vi "ParseObject.vi"(8 "error in (no error)":errorcluster, 10 "Index In":i32, 11 "JSON String":string) -> (0 "error out":errorcluster, 2 "Index Out":i32, 3 "JSON Tree":variant)   [LabVIEW 2013, in "i3-json.lvlib"]
doc: "Use this template to build a VI to use as a subVI."
uses:
  i3-json.lvlib
  JSON Types/JSON Type.ctl
  Token.ctl
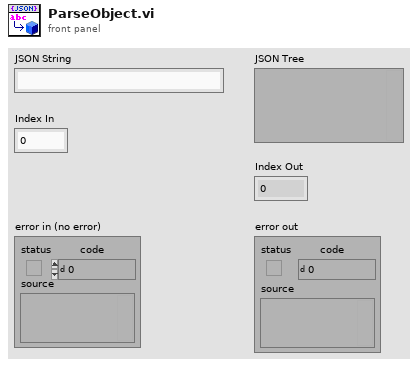
[diagram p1: front panel]
types:
  T1 = typedef "i3-json.lvlib/JSON Type.ctl" = enum8{"JSON Compatible", "JSON Array", "JSON Object", "JSON Null", "Double", "String", "Boolean", "Unknown"}
  T2 = typedef "i3-json.lvlib/Token.ctl" = enum16{"NONE", "CURLY_OPEN", "CURLY_CLOSE", "SQUARED_OPEN", "SQUARED_CLOSE", "COLON", "COMMA", "STRING", "NUMBER", "TRUE", "FALSE", "NULL"}
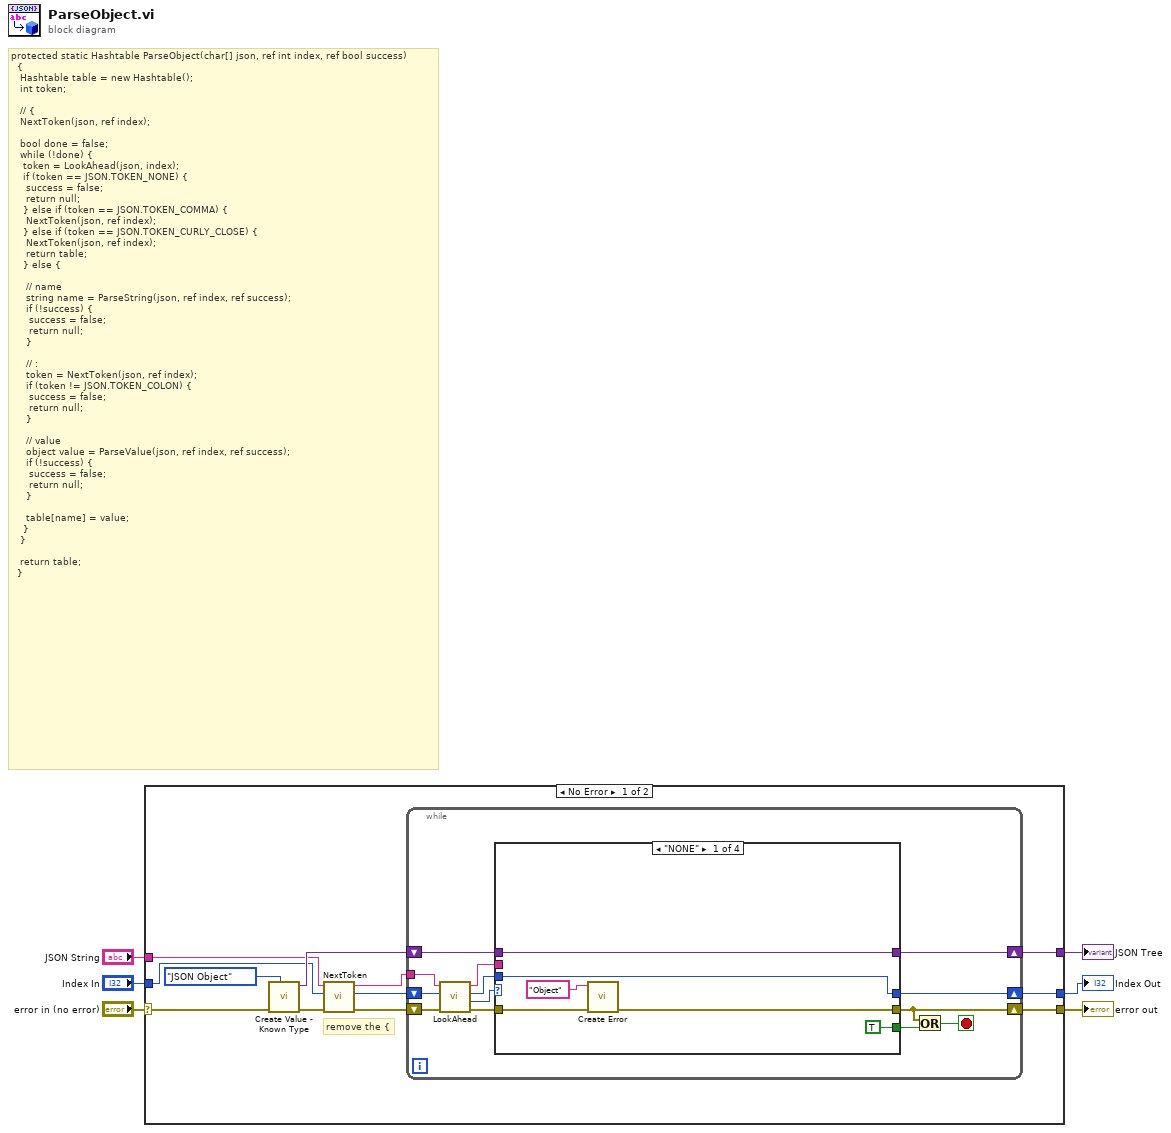
[diagram p0: block diagram]
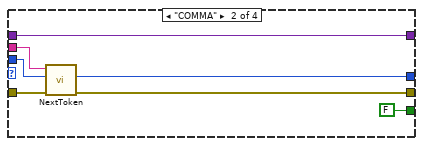
[diagram p2: hidden frame]
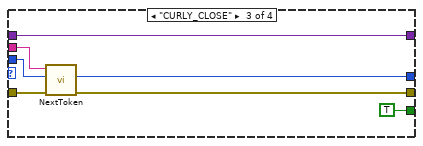
[diagram p3: hidden frame]
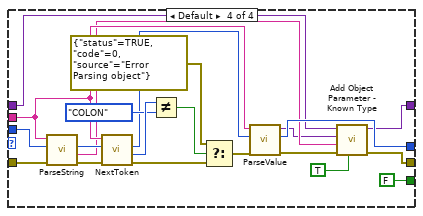
[diagram p4: hidden frame]
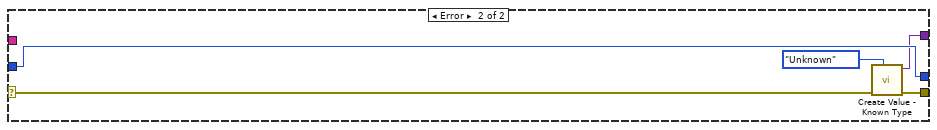
[diagram p5: hidden frame]
diagram:
  # "protected static Hashtable ParseObject(char[] json, ref int index, ref bool success)\n\t\t{\n\t\t\tHashtable table = new Hashtable();\n\t\t\tint token;\n\n\t\t\t// {\n\t\t\tNextToken(json, ref index);\n\n\t\t\tbool done = false;\n\t\t\twhile (!done) {\n\t\t\t\ttoken = LookAhead(json, index);\n\t\t\t\tif (token == JSON.TOKEN_NONE) {\n\t\t\t\t\tsuccess = false;\n\t\t\t\t\treturn null;\n\t\t\t\t} else if (token == JSON.TOKEN_COMMA) {\n\t\t\t\t\tNextToken(json, ref index);\n\t\t\t\t} else if (token == JSON.TOKEN_CURLY_CLOSE) {\n\t\t\t\t\tNextToken(json, ref index);\n\t\t\t\t\treturn table;\n\t\t\t\t} else {\n\n\t\t\t\t\t// name\n\t\t\t\t\tstring name = ParseString(json, ref index, ref success);\n\t\t\t\t\tif (!success) {\n\t\t\t\t\t\tsuccess = false;\n\t\t\t\t\t\treturn null;\n\t\t\t\t\t}\n\n\t\t\t\t\t// :\n\t\t\t\t\ttoken = NextToken(json, ref index);\n\t\t\t\t\tif (token != JSON.TOKEN_COLON) {\n\t\t\t\t\t\tsuccess = false;\n\t\t\t\t\t\treturn null;\n\t\t\t\t\t}\n\n\t\t\t\t\t// value\n\t\t\t\t\tobject value = ParseValue(json, ref index, ref success);\n\t\t\t\t\tif (!success) {\n\t\t\t\t\t\tsuccess = false;\n\t\t\t\t\t\treturn null;\n\t\t\t\t\t}\n\n\t\t\t\t\ttable[name] = value;\n\t\t\t\t}\n\t\t\t}\n\n\t\t\treturn table;\n\t\t}"
  n1 = case shown="No Error" "error in (no error)" {
    selector: "error in (no error)" -> [w18 w75]
    tunnel: [w15 w76] -> w5
    tunnel: "Index In" -> [w10 w77]
    tunnel: [w13 w77] -> w3
    tunnel: [w14 w74] -> w2
    tunnel: "JSON String" -> [w7 _]
    frame No Error {
      # "remove the {"
      n2 = call "Create Value - Known Type.vi"("JSON Type"=JSON_Type."JSON Object", "error in (no error)"=w18) -> ("error out"=w9:errorcluster, "JSON Tree"=w16:variant)  [unwired: 8 in]
      n3 = call "NextToken.vi"("error in (no error)"=w9, "Index In"=w10, "JSON String"=w7) -> ("error out"=w12:errorcluster, "Index Out"=w11:i32, "JSON String Passthrough"=w8:string)  [unwired: 4 in, 1 out]
      n4 = while {
        tunnel: w8 -> [w30]
        shift-right: [w25] -> w13
        shift-left: w11 -> [w29]
        shift-right: [w22] -> w14
        shift-left: w16 -> [w23]
        shift-right: [w19] -> w15
        shift-left: w12 -> [w31]
        stop <- w20 stop-if-true
        n5 = call "LookAhead.vi"("error in (no error)"=w31, "Index"=w29, "JSON String"=w30) -> ("error out"=w27:errorcluster, "TOKEN"=w28:T2, "Index Passthrough"=w26:i32, "JSON String Passthrough"=w24:string)  [unwired: 4 in]
        n6 = case shown="\"NONE\"" w28 {
          tunnel: [TRUE FALSE TRUE FALSE] -> w21
          tunnel: w27 -> [w33 w44 w51 w72]
          tunnel: [w32 w41 w48 w58] -> w19
          tunnel: w26 -> [w36 w43 w50 w71]
          tunnel: [w36 w42 w49 w60] -> w25
          tunnel: w24 -> [_ w38 w45 w62]
          tunnel: w23 -> [w35 w39 w46 w53]
          tunnel: [w35 w39 w46 w54] -> w22
          frame "NONE" {
            n7 = call "Create Error.vi"("error in (no error)"=w33, "datatype"="Object") -> ("error out"=w32:errorcluster)  [unwired: 9 in]
          }
          frame "COMMA" {
            n8 = call "NextToken.vi"("error in (no error)"=w44, "Index In"=w43, "JSON String"=w38) -> ("error out"=w41:errorcluster, "Index Out"=w42:i32)  [unwired: 4 in, 2 out]
          }
          frame "CURLY_CLOSE" {
            n9 = call "NextToken.vi"("error in (no error)"=w51, "Index In"=w50, "JSON String"=w45) -> ("error out"=w48:errorcluster, "Index Out"=w49:i32)  [unwired: 4 in, 2 out]
          }
          frame Default {
            n10 = call "ParseString.vi"("error in (no error)"=w72, "Index In"=w71, "JSON String"=w62) -> ("error out"=w70:errorcluster, "Parsed String"=w57:string, "Index Out"=w69:i32)  [unwired: 5 in, 1 out]
            n11 = call "NextToken.vi"("error in (no error)"=w70, "Index In"=w69, "JSON String"=w62) -> ("error out"=w65:errorcluster, "TOKEN"=w68:T2, "Index Out"=w61:i32)  [unwired: 4 in, 1 out]
            n12 = Not Equal?(x=w68, y=Token."COLON") -> (x != y?=w66:bool)
            n13 = Select(t=errorcluster {"status"=TRUE, "code"=0, "source"="Error Parsing object"}, s=w66, f=w65) -> (s? t:f=w63:errorcluster)
            n14 = call "ParseValue.vi"("error in (no error)"=w63, "Index In"=w61, "JSON String"=w62) -> ("error out"=w59:errorcluster, "Index Out"=w60:i32, "JSON Tree"=w55:variant)  [unwired: 6 in]
            n15 = call "Add Object Parameter - Known Type.vi"("Add Parameter as JSON Tree?"=TRUE ("Add Parameter\n as JSON Tree?"), "error in (no error)"=w59, "Name"=w57, "Value"=w55, "JSON Tree in (JSON Object)"=w53) -> ("error out"=w58:errorcluster, "JSON Tree out (JSON Object)"=w54:variant)  [unwired: 5 in]
          }
        }
        n16 = Or(x=w19, y=w21) -> (x .or. y?=w20:bool)
      }
    }
    frame Error {
      n17 = call "Create Value - Known Type.vi"("JSON Type"=JSON_Type."Unknown", "error in (no error)"=w75) -> ("error out"=w76:errorcluster, "JSON Tree"=w74:variant)  [unwired: 8 in]
    }
  }
  "error out" <- w5
  "JSON Tree" <- w2
  "Index Out" <- w3
